vi "pl1000GetValues.vi"(0 "pl1000 handle":i16, 5 "noOfValues":u32, 7 "SizeOfArray":u32, 11 "error in (no error)":errorcluster) -> (4 "pl1000 handle out":i16, 6 "values":u16[](array[numeric]), 8 "Ch Over Range":bool[](array[boolean]), 10 "noOfValues collected per ch":u32, 14 "triggerIndex":u32, 15 "error out":errorcluster)   [LabVIEW 2010]
doc: "This function is used to get values after calling pl1000Run \n\nvalues: an array of sample values returned by the function. The size of this buffer must be the number of enabled channels multiplied by the number of samples to be collected.\n\nnoOfValues: the number of sample values per channel that the function should collect. \n\nnOfChannels: the number of channels the device is configured to read data from.\n\noverflow: a bit field indicating which, if any, input channels overflowed the input range of the device. A bit set to 1 indicates an overflow. The least significant bit corresponds to channel 1. May be NULL if an overflow warning is not required. \n\nnoOfValues collecetd: the number of samples per channel that were actually written to the buffer. \n\ntriggerIndex: a number indicating when the trigger event occurred. The number is a zero-based index to the values array, or 0xFFFFFFFF if the information is not available."
uses:
  pl1000.dll
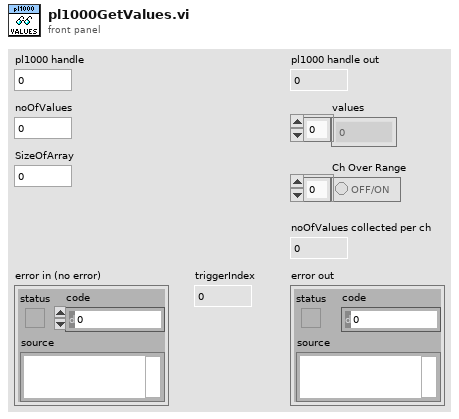
[diagram p1: front panel]
types:
  T1 = cluster{"status":bool, "code":u32, "source":string}
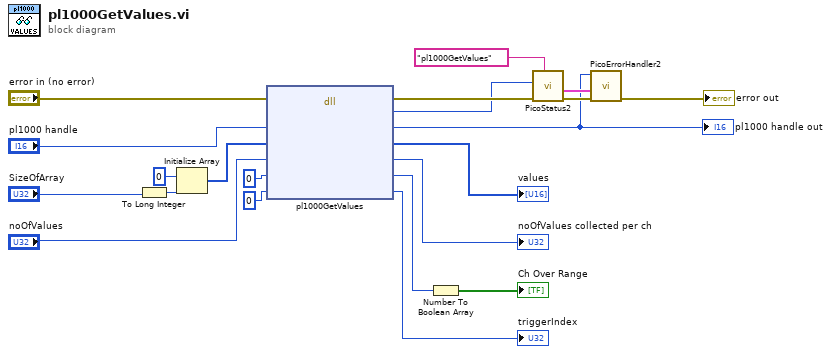
[diagram p0: block diagram]
diagram:
  n1 = To Long Integer(number="SizeOfArray") -> (32bit integer=w4:i32)
  n2 = Initialize Array(u16 0, w4) -> (w13:u16[])
  n3 = dll-call lib="pl1000.dll" fn="pl1000GetValues"(error in="error in (no error)", "handle"="pl1000 handle", "values"=w13, "noOfValues"="noOfValues", "overflow"=u16 0, "triggerIndex"=u32 0) -> (error out=w8:errorcluster, "status"=w7:u32, "handle"=w5:i16, "values"=→"values":u16[], "noOfValues"=→"noOfValues collected per ch":u32, "overflow"=w19:u16, "triggerIndex"=→"triggerIndex":u32)  [unwired: 2 in, 1 out]
  "pl1000 handle out" <- w5
  n4 = Number To Boolean Array(number=w19) -> (Boolean array=→"Ch Over Range":bool[])
  n5 = call "PicoStatus2.vi"("PICO source"="pl1000GetValues", "Error in"=w8, "PICO STATUS"=w7) -> ("error out"=w11:errorcluster, "PICO_STATUS out"=w10:T1)  [unwired: 5 in]
  n6 = call "PicoErrorHandler2.vi"("error in (no error)"=w11, "PICO_STATUS in"=w10, "handle In"=w5) -> ("error out"=→"error out":errorcluster)  [unwired: 8 in]
